vi "降采样.vi"() -> ()   [LabVIEW 2012]
uses:
  <vilib>/Analysis/2dsp.llb/Decimate (continuous, DBL).vi
  <vilib>/measure/NI_MABase.lvlib
  <vilib>/Analysis/NI_AALPro.lvlib
panel:
  in  "decimating factor":i32=100 caption="降采样因子"
  in  "frequency":dbl=4.0 caption="频率" format="%0.2p"
  out "波形图":waveform(dbl)[](graph)=[{"t0"=timestamp(2160.2791 s since 1904-01-01), "dt"=0.0001, "Y"=array[10000 elements]}, {"t0"=timestamp(2160.2791 s since 1904-01-01), "dt"=0.01, "Y"=[3.684547105929593, 3.8443279255026797, 3.9510565162955364, 3.99802672842835, 3.982287250728456, 3.9048270524654916, 3.7705132427749994, 3.5877852522914706, 3.368124552683526, 3.1253332335630746, 2.874666766434466, 2.6318754473141697, 2.4122147477065243, 2.2294867572234205, 2.095172947533453, 2.0177127492710785, 2.0019732715718055, 2.0489434837052287, 2.1556720744986477, 2.3154528940722137, 2.518246325899369, 2.751310112836344, 3.000000000001238, 3.248689887166054, 3.4817536741028006, 3.6845471059295916, 3.844327925502679, 3.9510565162955373, 3.998026728428351, 3.982287250728459, 3.904827052465494, 3.7705132427750017, 3.5877852522914733, 3.3681245526835286, 3.1253332335630772, 2.8746667664344683, 2.631875447314171, 2.4122147477065248, 2.2294867572234214, 2.095172947533452, 2.0177127492710776, 2.0019732715718033, 2.048943483705226, 2.155672074498645, 2.3154528940722106, 2.5182463258993666, 2.7513101128363417, 3.0000000000012363, 3.2486898871660532, 3.4817536741028, 3.684547105929592, 3.8443279255026805, 3.951056516295539, 3.998026728428353, 3.982287250728461, 3.904827052465497, 3.7705132427750048, 3.587785252291476, 3.3681245526835304, 3.1253332335630786, 2.874666766434469, 2.631875447314171, 2.4122147477065243, 2.2294867572234196, 2.09517294753345, 2.0177127492710754, 2.001973271571801, 2.0489434837052234, 2.1556720744986424, 2.3154528940722083, 2.518246325899365, 2.751310112836341, 3.0000000000012355, 3.248689887166053, 3.4817536741028006, 3.6845471059295933, 3.8443279255026814, 3.951056516295541, 3.998026728428355, 3.9822872507284632, 3.904827052465499, 3.7705132427750065, 3.5877852522914777, 3.3681245526835317, 3.1253332335630795, 2.874666766434469, 2.631875447314171, 2.412214747706524, 2.2294867572234183, 2.095172947533449, 2.017712749271073, 2.001973271571799, 2.048943483705221, 2.1556720744986406, 2.3154528940722066, 2.518246325899364, 2.75131011283634, 3.0000000000012355, 3.2486898871660532, 3.4817536741028015]}]
  in  "sampling info":cluster{"Fs":dbl, "#s":dbl}={"Fs"=10000.0, "#s"=10000.0} caption="采样信息" {"Fs" format="%.2p"}
  in  "停止":bool
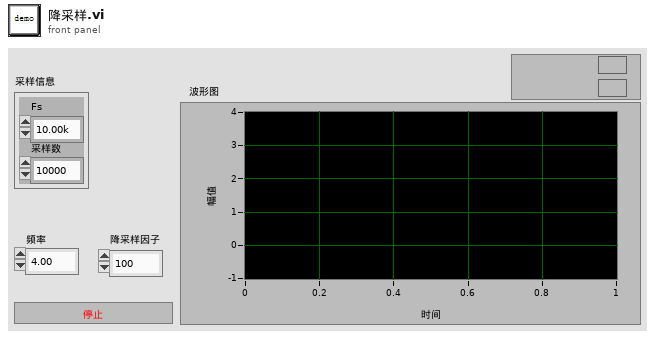
[diagram p1: front panel]
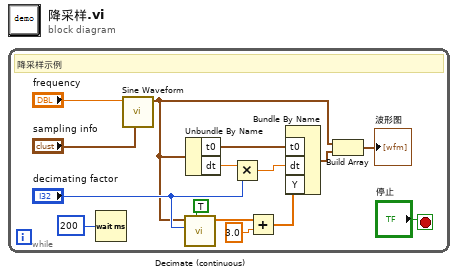
[diagram p0: block diagram]
diagram:
  n1 = while {
    stop <- "停止" stop-if-true
    # "降采样示例"
    n2 = Wait (ms)(milliseconds to wait=u32 200 ("等待时间（毫秒）")) -> ()  [unwired: 1 out]
    n3 = call <vilib>:"Sine Waveform.vi"("sampling info"="sampling info", "frequency"="frequency") -> ("signal out"=w3:waveform(dbl))  [unwired: 8 in, 1 out]
    n4 = call-poly <vilib>:"Decimate (continuous).vi"("reset"=TRUE, "decimating factor"="decimating factor", "X"=w3) -> ("Decimated Array"=w6:dbl[])  [unwired: 7 in, 1 out]
    n5 = Unbundle By Name(w3) -> ("t0"=w7:timestamp, "dt"=w10:dbl)
    n6 = Multiply(x=w10, y="decimating factor") -> (x*y=w8:dbl)
    n7 = Add(x=w6, y=3.0) -> (x+y=w4:dbl[])
    n8 = Bundle By Name("t0"=w7, "dt"=w8, "Y"=w4) -> (w2:waveform(dbl))  [unwired: 1 in]
    n9 = Build Array(w3, w2) -> (→"波形图":waveform(dbl)[])
  }
